vi "Virtual Camera Finish Stream.vi"(5 "Frames to Skip":u32, 6 "Shutter to Open":T2=enum."Cy3 (532 nm)", 7 "Auto Shutter":bool, 8 "error in (no error)":errorcluster, 9 "Camera Settings":T1={"Exposure Time (ms)"=100.0, "Binning"=enum."2x2", "Scan Mode (Flash)"=enum."Fast", "Trigger Mode (Flash)"=enum."Fast", "Frames to Acquire"=1000.0, "Pixel Correction (Flash)"=FALSE} {"Exposure Time (ms)" min=1.0 max=10000.0 step=1.0}, 10 "File Path":path, 11 "Virtual Camera in":refnum<class "Virtual Camera.lvclass">) -> (0 "error out":errorcluster, 3 "Virtual Camera out":refnum<class "Virtual Camera.lvclass">)   [LabVIEW 2017, in "Virtual Camera.lvlib" / "Virtual Camera.lvclass"]
uses:
  Virtual Camera.lvclass
  C:/Program Files/National Instruments/LabVIEW 2017/vi.lib/ActorFramework/Actor/Actor.lvclass
  Resources/Type Defs/Excitation.ctl
  Resources/Type Defs/Camera Settings.ctl
  Virtual Camera.lvclass/Virtual Camera.ctl
  <vilib>/ActorFramework/Message Enqueuer/Message Enqueuer.lvclass/Message Enqueuer.ctl
  <vilib>/ActorFramework/Actor/Actor.lvclass/Actor.ctl
  Application Messages/Close Shutter Msg/Close Shutter Msg.lvclass/Close Shutter Msg.ctl
  BinaryTIFF v0.3.2b/Class/TIFF.lvclass
  <vilib>/ActorFramework/Message Enqueuer/Enqueue.vi
  <vilib>/ActorFramework/Stop Msg/Stop Msg.lvclass
  C:/Program Files/National Instruments/LabVIEW 2017/vi.lib/ActorFramework/Message/Message.lvclass
  Orca-Flash 4.0 V2 Messages/Flash Finish Stream Msg/Flash Finish Stream Msg.lvclass
  Application Messages/Close Shutter Msg/Close Shutter Msg.lvclass
  Resources/GLOBAL/GLOBAL Time-critical.vi
  <vilib>/ActorFramework/Message Priority Queue/Priority Enqueue.vi
  <vilib>/ActorFramework/Actor/Actor.lvclass
  kernel32.dll
  BinaryTIFF v0.3.2b/CLib/DCIMG2TIFF/x64/Release/dcimg2tiff.dll
panel:
  in  "Stop Button":bool
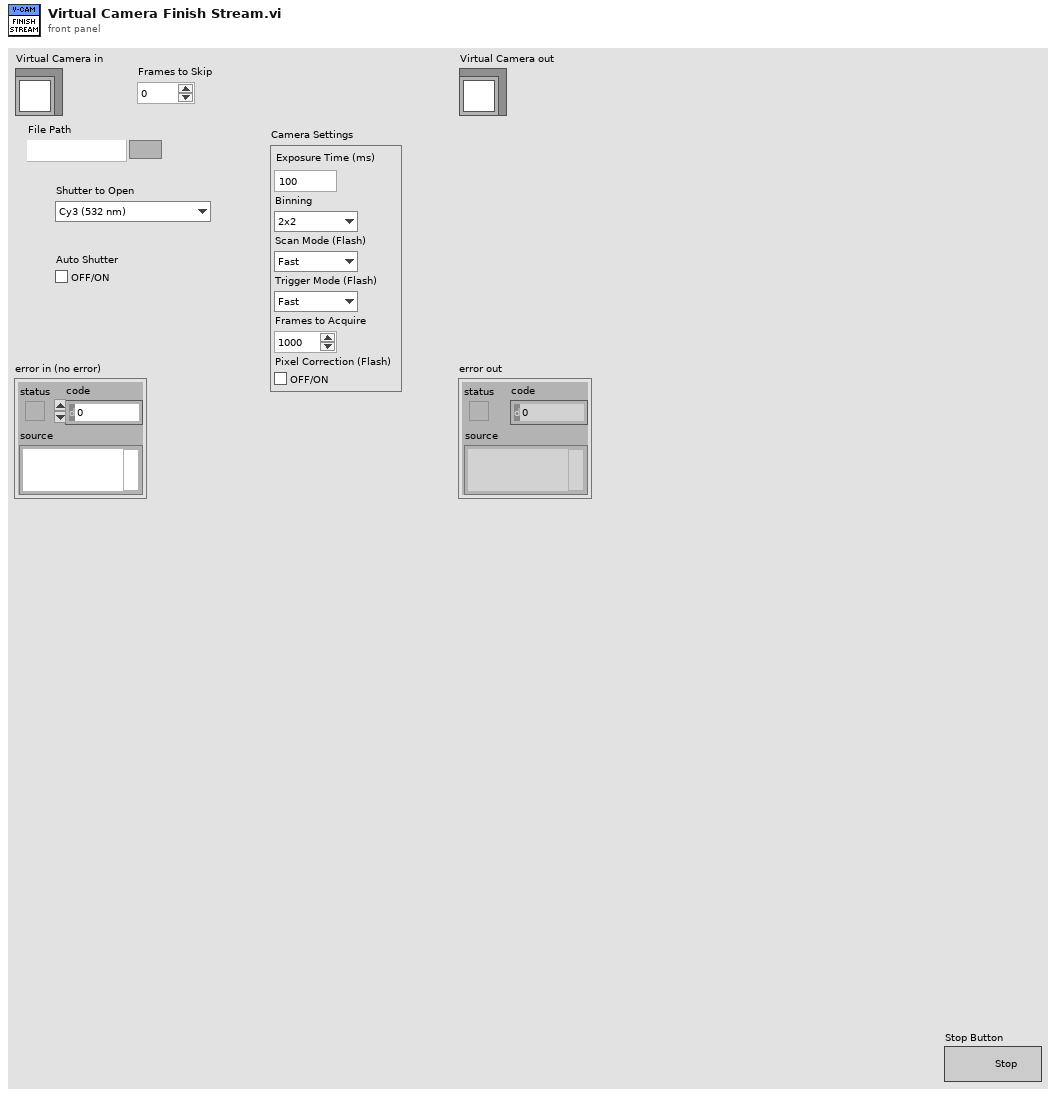
[diagram p1: front panel]
types:
  T1 = typedef "Camera Settings.ctl" = cluster{"Exposure Time (ms)":dbl, "Binning":enum16{"1x1", "2x2", "4x4"}, "Scan Mode (Flash)":enum16{"Fast", "Slow"}, "Trigger Mode (Flash)":enum16{"Fast", "Standard"}, "Frames to Acquire":dbl, "Pixel Correction (Flash)":bool}
  T2 = typedef "Excitation.ctl" = enum16{"Cy2 (473 nm)", "Cy3 (532 nm)", "Cy5 (639 nm)", "Cy7 (730 nm)", "Cy2/Cy3", "Cy3/Cy5", "Cy3/Cy7", "Cy5/Cy7"}
  T3 = enum16{"<unknown>", "Evolve 512", "Orca-Flash 4.0 V2"}
  T4 = cluster{"Number of Frames":u32, "Image Width (px)":u32, "Image Height (px)":u32, "Pixel Size (nm)":dbl, "Exposure Time (ms)":dbl, "Frame Time (ms)":dbl, "Number of Channels":u32, "Camera Type":enum16{"<unknown>", "Evolve 512", "Orca-Flash 4.0 V2"}, "Bit Depth":u32, "Image Description":string}
  T5 = typedef "Physical Camera Assignment.ctl" = cluster{"Channel Name":string, "Camera Type":T6, "Serial Number":string, "Flip Vertically":bool, "Flip Horizontally":bool}
  T6 = typedef "Camera Type.ctl" = enum16{"Orca-Flash 4.0 V2"}
  T7 = cluster{"appended path":path, "Flip Vertically":bool, "Flip Horizontally":bool}[]
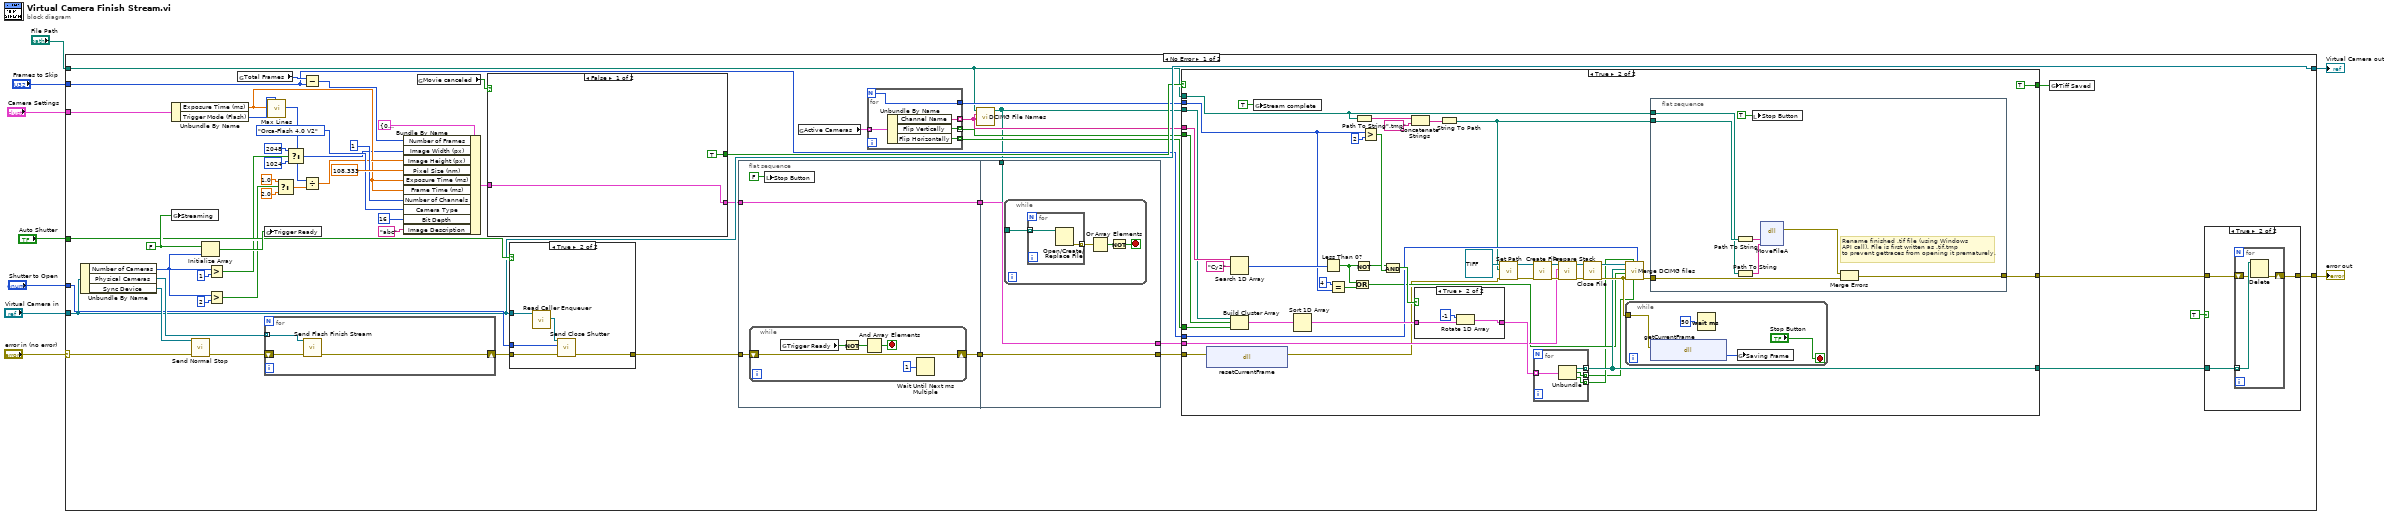
[diagram p0: block diagram]
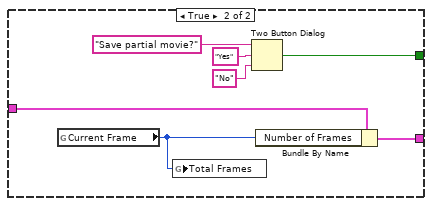
[diagram p3: hidden frame]
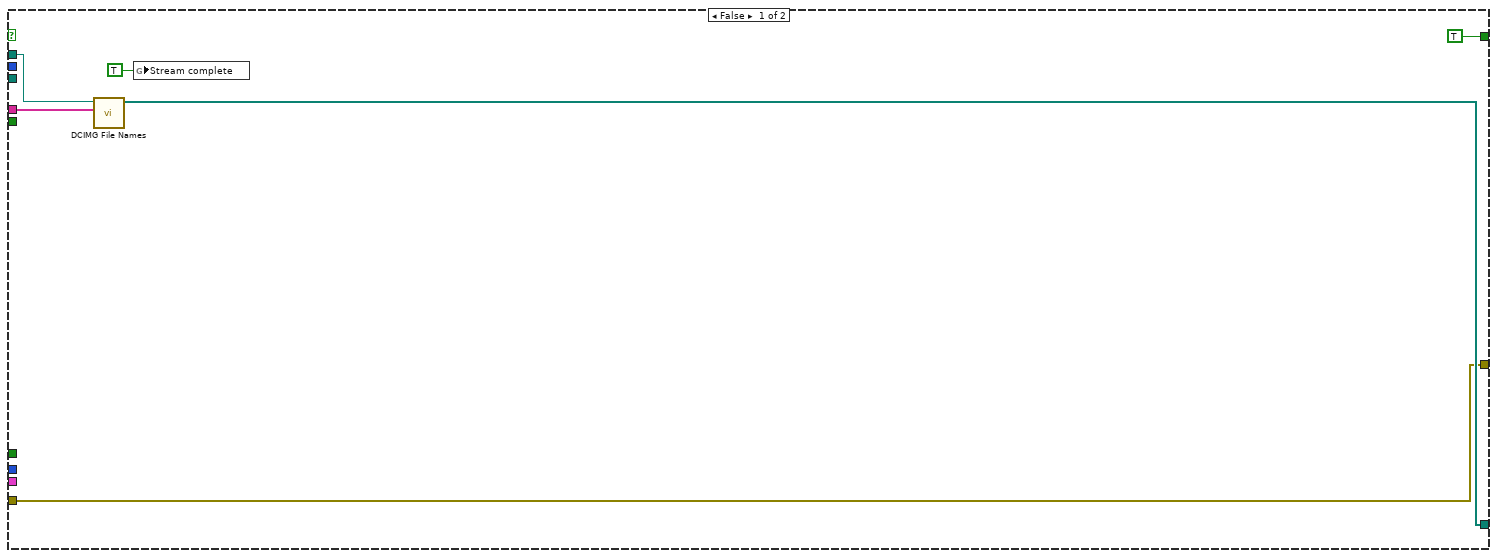
[diagram p4: hidden frame]
diagram:
  n1 = case shown="No Error" "error in (no error)" {
    selector: "error in (no error)" -> [w63 w184]
    tunnel: [w42 w184] -> w8
    tunnel: [w48 w183] -> w6
    tunnel: "Virtual Camera in" -> [w48 w183]
    tunnel: "Auto Shutter" -> [w59 _]
    tunnel: "Shutter to Open" -> [w57 _]
    tunnel: "File Path" -> [w19 _]
    tunnel: "Camera Settings" -> [w55 _]
    tunnel: "Frames to Skip" -> [w29 _]
    frame No Error {
      w61 = FALSE
      n2 = Unbundle By Name(w48) -> ("Number of Cameras"=w17:i32, "Physical Cameras"=w65:refnum<class "Message Enqueuer.lvclass">[], "Sync Device"=w64:refnum<class "Message Enqueuer.lvclass">)
      n3 = Unbundle By Name(w55) -> ("Exposure Time (ms)"=w43:dbl, "Trigger Mode (Flash)"=w45:enum16{"Fast", "Standard"})
      n4 = global write "GLOBAL Time-critical.vi" "Streaming"(w61) -> ()
      n5 = call <vilib>:"Send Normal Stop.vi"("error in (no error)"=w63, "Message Enqueuer"=w64) -> ("error out"=w60:errorcluster)  [unwired: 9 in]
      n6 = Initialize Array(w61, w17) -> (w62:bool[])
      n7 = Greater?(x=w17, y=1) -> (0:w15:bool)
      n8 = Greater?(x=w17, y=2) -> (0:w38:bool)
      n9 = global read "GLOBAL Time-critical.vi" "Total Frames"() -> (w30:i32)
      n10 = global write "GLOBAL Time-critical.vi" "Trigger Ready"(w62) -> ()
      n11 = for {
        tunnel: w65 -> [w182] mode=indexing
        shift-right: [w181] -> w58
        shift-left: w60 -> [w180]
        n12 = call "Send Flash Finish Stream.vi"("error in (no error)"=w180, "Message Enqueuer"=w182) -> ("error out"=w181:errorcluster)  [unwired: 8 in, 1 out]
      }
      n13 = call "Max Lines.vi"("Trigger Mode"=w45, "Frame Time (ms)"=w43) -> ("Max Lines"=w46:i32)  [unwired: 8 in, 1 out]
      n14 = Select(t=1.0, s=w38, f=2.0) -> (s? t:f=w39:dbl)
      n15 = Select(t=u32 2048 ("Image Width (px)"), s=w15, f=u32 1024) -> (s? t:f=w13:u32)
      n16 = Subtract(x=w30, y=w29) -> (x-y=w28:u32)
      n17 = Divide(x=w46, y=w39) -> (x/y=w44:dbl)
      n18 = Bundle By Name(cluster=T4 {"Number of Frames"=0, "Image Width (px)"=0, "Image Height (px)"=0, "Pixel Size (nm)"=0.0, "Exposure Time (ms)"=0.0, "Frame Time (ms)"=0.0, "Number of Channels"=0, "Camera Type"=enum."<unknown>", "Bit Depth"=0, "Image Description"=""} ("Stack Info"), "Number of Frames"=w28, "Image Width (px)"=w13, "Image Height (px)"=w44, "Pixel Size (nm)"=108.333, "Exposure Time (ms)"=w43, "Frame Time (ms)"=w43, "Number of Channels"=u32 1, "Camera Type"=T3."Orca-Flash 4.0 V2", "Bit Depth"=u32 16, "Image Description"="abc") -> (w33:T4)
      n19 = global read "GLOBAL Time-critical.vi" "Movie canceled"() -> (w35:bool)
      n20 = case shown="False" w35 {
        tunnel: [TRUE ("T button?") w80] -> w34
        tunnel: w33 -> [w78 w83]
        tunnel: [w78 w82] -> w32
        frame False {
        }
        frame True {
          n21 = global read "GLOBAL Time-critical.vi" "Current Frame"() -> (w81:i32)
          n22 = global write "GLOBAL Time-critical.vi" "Total Frames"(w81) -> ()
          n23 = Two Button Dialog(message="Save partial movie?", 1:"No" ("F button name (\"Cancel\")"), 2:"Yes" ("T button name (\"OK\")")) -> (T button?=w80:bool)
          n24 = Bundle By Name(cluster=w83, "Number of Frames"=w81) -> (w82:T4)
        }
      }
      n25 = case shown="True" w59 {
        tunnel: w58 -> [w174 w176]
        tunnel: w48 -> [_ w179]
        tunnel: w57 -> [_ w177]
        tunnel: [w174 w175] -> w49
        frame False {
        }
        frame True {
          n26 = call <vilib>:"Read Caller Enqueuer.vi"("Actor"=w179) -> ("Caller Enqueuer"=w178:refnum<class "Message Enqueuer.lvclass">)  [unwired: 10 in]
          n27 = call "Send Close Shutter.vi"("error in (no error)"=w176, "Shutter to Close"=w177, "Message Enqueuer"=w178) -> ("error out"=w175:errorcluster)  [unwired: 7 in, 1 out]
        }
      }
      n28 = flat-sequence {
        tunnel: w49 -> [w159]
        tunnel: w32 -> [w156]
        tunnel: [w157] -> w27
        tunnel: [w156] -> w26
        tunnel: [w166] -> w31
        tunnel: [w167] -> w47
        tunnel: w27 -> [w167]
        tunnel: w26 -> [w166]
        tunnel: w18 -> [w165]
        frame #0 {
          n29 = while {
            shift-right: [w164] -> w157
            shift-left: w159 -> [w164]
            stop <- w163 stop-if-true
            n30 = global read "GLOBAL Time-critical.vi" "Trigger Ready"() -> (w161:bool[])
            n31 = Not(x=w161) -> (.not. x?=w160:bool[])
            n32 = And Array Elements(Boolean array=w160) -> (logical AND=w163:bool)
            n33 = Wait Until Next ms Multiple(millisecond multiple=u32 1) -> ()  [unwired: 1 out]
          }
          n34 = local write "Stop Button"(FALSE ("Stop Button")) -> ()
        }
        frame #1 {
          n35 = while {
            tunnel: w165 -> [w171]
            stop <- w169 stop-if-true
            n36 = for {
              tunnel: w171 -> [w172] mode=indexing
              tunnel: [w173] -> w170 mode=indexing
              n37 = Open/Create/Replace File(file path (use dialog)=w172) -> (error out=w173:errorcluster)  [unwired: 5 in, 2 out]
            }
            n38 = Or Array Elements(Boolean array=w170) -> (logical OR=w168:bool)
            n39 = Not(x=w168) -> (.not. x?=w169:bool)
          }
        }
      }
      n40 = global read "GLOBAL Time-critical.vi" "Active Cameras"() -> (w24:T5[])
      n41 = for {
        N -> [w73]
        tunnel: w24 -> [w77] mode=indexing
        tunnel: [w75] -> w23 mode=indexing
        tunnel: [w76] -> w22 mode=indexing
        tunnel: [w74] -> w20 mode=indexing
        tunnel: [w73] -> w21
        n42 = Unbundle By Name(w77) -> ("Channel Name"=w74:string, "Flip Vertically"=w75:bool, "Flip Horizontally"=w76:bool)
      }
      n43 = call "DCIMG File Names.vi"("Channel Names"=w20, "TIFF File Path"=w19) -> ("DCIMG Files"=w18:path[])  [unwired: 9 in]
      n44 = case shown="True" w34 {
        tunnel: w19 -> [w92 w112]
        tunnel: w47 -> [w89 w95]
        tunnel: w31 -> [_ w104]
        tunnel: [w89 w117] -> w41
        tunnel: [w91 w99] -> w11
        tunnel: w29 -> [_ w100]
        tunnel: [TRUE ("Tiff Saved") TRUE ("Tiff Saved")] -> w25
        tunnel: w21 -> [_ w122]
        tunnel: w22 -> [_ w121]
        tunnel: w23 -> [_ w120]
        tunnel: w20 -> [w88 w119]
        tunnel: w18 -> [_ w116]
        frame False {
          n45 = call "DCIMG File Names.vi"("Channel Names"=w88, "TIFF File Path"=w92) -> ("DCIMG Files"=w91:path[])  [unwired: 9 in]
          n46 = global write "GLOBAL Time-critical.vi" "Stream complete"(TRUE ("Stream complete")) -> ()
        }
        frame True {
          n47 = dll-call lib="C:/LVDEV/current microscope software/BinaryTIFF v0.3.2b/CLib/DCIMG2TIFF/x64/Release/dcimg2tiff.dll" fn="resetCurrentFrame"(error in=w95) -> (error out=w94:errorcluster)  [unwired: 3 in, 1 out]
          n48 = Build Cluster Array(w116, w120, w121) -> (w126:T7)
          n49 = Search 1D Array(1D array=w119, element="Cy2") -> (index of element=w134:i32)  [unwired: 1 in]
          n50 = global write "GLOBAL Time-critical.vi" "Stream complete"(TRUE ("Stream complete")) -> ()
          n51 = Sort 1D Array(array=w126) -> (sorted array=w133:T7)
          n52 = Less Than 0?(x=w134) -> (x < 0?=w129:bool)
          n53 = Equal?(x=4, y=w122) -> (x = y?=w128:bool)
          n54 = Or(x=w129, y=w128) -> (x .or. y?=w98:bool)
          n55 = Path To String(path=w112) -> (string=w115:string)
          n56 = Not(x=w129) -> (.not. x?=w124:bool)
          n57 = Greater?(x=w122, y=2) -> (0:w131:bool)
          n58 = And(x=w124, y=w131) -> (x .and. y?=w130:bool)
          n59 = Concatenate Strings(w115, ".tmp" ("string")) -> (w113:string)
          n60 = case shown="True" w130 {
            tunnel: w133 -> [w140 w143]
            tunnel: [w140 w142] -> w125
            frame False {
            }
            frame True {
              n61 = Rotate 1D Array(1:w143, 2:-1 ("n")) -> (0:w142:T7)
            }
          }
          n62 = String To Path(string=w113) -> (path=w93:path)
          n63 = call-dynamic "Set Path.vi"("error in (no error)"=w94, "File Path"=w93, "TIFF in"=refnum<class "TIFF.lvclass"> refnum ("BinaryTIFF.lvlib:TIFF.lvclass")) -> ("error out"=w111:errorcluster, "TIFF out"=w107:refnum<class "TIFF.lvclass">)  [unwired: 7 in]
          n64 = call-dynamic "Create File.vi"("error in (no error)"=w111, "TIFF in"=w107) -> ("error out"=w110:errorcluster, "TIFF out"=w106:refnum<class "TIFF.lvclass">)  [unwired: 8 in]
          n65 = for {
            tunnel: w125 -> [w139] mode=indexing
            tunnel: [w138] -> w99 mode=indexing
            tunnel: [w137] -> w96 mode=indexing
            tunnel: [w136] -> w97 mode=indexing
            n66 = Unbundle(w139) -> ("appended path"=w138:path, "Flip Vertically"=w137:bool, "Flip Horizontally"=w136:bool)
          }
          n67 = call-dynamic "Prepare Stack.vi"("error in (no error)"=w110, "Stack Info"=w104, "TIFF in"=w106) -> ("error out"=w109:errorcluster, "TIFF out"=w105:refnum<class "TIFF.lvclass">)  [unwired: 7 in]
          n68 = call-dynamic "Close File.vi"("error in (no error)"=w109, "TIFF in"=w105) -> ("error out"=w102:errorcluster, "TIFF out"=w103:refnum<class "TIFF.lvclass">)  [unwired: 8 in]
          n69 = call-dynamic "Merge DCIMG files.vi"("Frames to Skip"=w100, "Horizontal Flip"=w96, "Vertical Flip"=w97, "error in (no error)"=w102, "Channel 3 Right?"=w98, "DCIMG Paths (2 to 4)"=w99, "TIFF in"=w103) -> ("error out"=w101:errorcluster)  [unwired: 3 in, 1 out]
          n70 = while {
            tunnel: w102 -> [w153]
            stop <- "Stop Button" stop-if-true
            n71 = dll-call lib="C:/LVDEV/current microscope software/BinaryTIFF v0.3.2b/CLib/DCIMG2TIFF/x64/Release/DCIMG2TIFF.dll" fn="getCurrentFrame"(error in=w153) -> ("Current Frame"=w152:u64)  [unwired: 2 in, 2 out]
            n72 = Wait (ms)(milliseconds to wait=u32 50) -> ()  [unwired: 1 out]
            n73 = global write "GLOBAL Time-critical.vi" "Saving Frame"(w152) -> ()
          }
          n74 = flat-sequence {
            tunnel: w101 -> [w147]
            tunnel: [w146] -> w117
            tunnel: w93 -> [w149]
            tunnel: w112 -> [w144]
            frame #0 {
              # "Rename finished .tif file (using Windows\nAPI call). File is first written as .tif.tmp\nto prevent gettraces from opening it prematurely."
              n75 = Path To String(path=w149) -> (string=w150:string)
              n76 = Path To String(path=w144) -> (string=w145:string)
              n77 = local write "Stop Button"(TRUE ("Stop Button")) -> ()
              n78 = dll-call lib="kernel32.dll" fn="MoveFileA"("arg1"=w150, "arg2"=w145) -> (error out=w148:errorcluster)  [unwired: 6 in, 1 out]
              n79 = Merge Errors(w148, w147) -> (w146:errorcluster)
            }
          }
        }
      }
      n80 = global write "GLOBAL Time-critical.vi" "Tiff Saved"(w25) -> ()
      n81 = case shown="True" TRUE {
        tunnel: [w66 w69] -> w42
        tunnel: w41 -> [w66 w68]
        tunnel: w11 -> [_ w67]
        frame False {
        }
        frame True {
          n82 = for {
            shift-right: [w70] -> w69
            shift-left: w68 -> [w71]
            tunnel: w67 -> [w72] mode=indexing
            n83 = Delete(path (use dialog)=w72, error in=w71) -> (error out=w70:errorcluster)  [unwired: 3 in, 2 out]
          }
        }
      }
    }
    frame Error {
    }
  }
  "error out" <- w8
  "Virtual Camera out" <- w6
